vi "Py Object I32.vi"(8 "error in (no error)":errorcluster) -> (0 "error out":errorcluster)   [LabVIEW 2020]
uses:
  G-Embedded-Python-Interpreter-Toolkit/Merge Call Library Errors.vi
  <vilib>/addons/_JKI Toolkits/Caraya/classes/Assert/Assert Not Error.vi
  <vilib>/addons/_JKI Toolkits/Caraya/classes/Assert/Assert Equal Value and Type_Variant.vi
  G-Embedded-Python-Interpreter-Toolkit/G-Embedded-Python-Interpreter-Toolkit.lvlib
  <vilib>/addons/_JKI Toolkits/Caraya/classes/Assert/Assert.lvclass
  <vilib>/addons/_JKI Toolkits/Caraya/classes/Test/Test.lvclass
panel:
  out "Value":i32
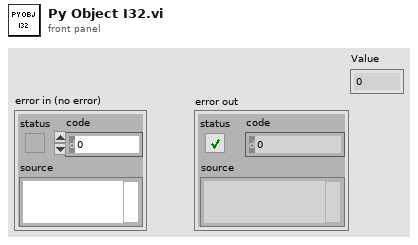
[diagram p1: front panel]
types:
  T1 = typedef "G-Embedded-Python-Interpreter-Toolkit.lvlib/Python Object Reference.ctl" = refnum<k1>
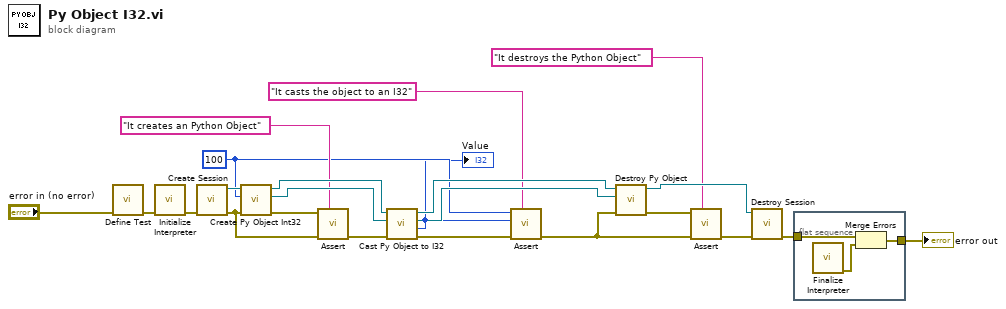
[diagram p0: block diagram]
diagram:
  w7 = 100 ("Value")
  n1 = call <vilib>:"Define Test.vi"("error in (no error)"="error in (no error)") -> ("error out"=w23:errorcluster)  [unwired: 10 in]
  n2 = call "Initialize Interpreter.vi"("error in (no error)"=w23) -> ("error out"=w20:errorcluster)  [unwired: 9 in, 1 out]
  n3 = call "Create Session.vi"("error in (no error)"=w20) -> ("error out"=w11:errorcluster, "Session Handle"=w19:refnum<data-value>)  [unwired: 9 in]
  n4 = call "Create Py Object Int32.vi"("error in (no error)"=w11, "Value"=w7, "Session Handle in"=w19) -> ("error out"=w12:errorcluster, "Python Object Refnum"=w17:T1, "Session Handle out"=w18:refnum<data-value>)  [unwired: 6 in]
  n5 = call-poly <vilib>:"Assert.vi"("Label"="It creates an Python Object", "error in (no error)"=w11, "Not Error?"=w12) -> ("error out"=w10:errorcluster)  [unwired: 8 in]
  n6 = call "Cast Py Object to I32.vi"("error in (no error)"=w10, "Python Object Refnum in"=w17, "Session Handle in"=w18) -> ("error out"=w8:errorcluster, "Value"=w6:i32, "Python Object Refnum out"=w16:T1, "Session Handle out"=w15:refnum<data-value>)  [unwired: 5 in]
  "Value" <- w6
  n7 = call-poly <vilib>:"Assert.vi"("Label"="It casts the object to an I32", "error in (no error)"=w8, "Y"=w6, "X"=w7) -> ("error out"=w3:errorcluster)  [unwired: 7 in]
  n8 = call "Destroy Py Object.vi"("error in (no error)"=w3, "Python Object Refnum"=w16, "Session Handle in"=w15) -> ("error out"=w4:errorcluster, "Session Handle out"=w14:refnum<data-value>)  [unwired: 7 in]
  n9 = call-poly <vilib>:"Assert.vi"("Label"="It destroys the Python Object", "error in (no error)"=w3, "Not Error?"=w4) -> ("error out"=w2:errorcluster)  [unwired: 8 in]
  n10 = call "Destroy Session.vi"("error in (no error)"=w2, "Session Handle"=w14) -> ("error out"=w13:errorcluster)  [unwired: 9 in]
  n11 = flat-sequence {
    tunnel: [w25] -> w21
    tunnel: w13 -> [w24]
    frame #0 {
      n12 = call "Finalize Interpreter.vi"() -> ("error out"=w26:errorcluster)  [unwired: 11 in]
      n13 = Merge Errors(w24, w26) -> (w25:errorcluster)
    }
  }
  "error out" <- w21
